vi "CRYDataView Curve Close.vi"   [LabVIEW 2013]
uses:
  CRYNew View Global.vi
types:
  T1 = typedef "Graph Main Info Cluster.ctl" = cluster{"Selected_BarIdx":i32, "Selected_PanelIdx":i32, "Graph Main VIRef":refnum<vi>, "ToolBarClick":bool, "Spliter Ref Array":refnum<vi>[], "Panel Ref Array":refnum<vi>[], "Spliter_matrix":i32[][], "Panel_matrix":i32[][], "child_spliterIdx_matrix":i32[][], "split_pos_matrix":i32[][], "Title State":bool, "sQueueName":string, "Frame nID":i32, "Graph VIRef Array":cluster{"Graph VIRef":refnum<vi>, "Panel Idx":i32, "Frame VIRef":refnum<vi>, "Icon Ring":i32, "Graph Type":string}[], "View Type":string}
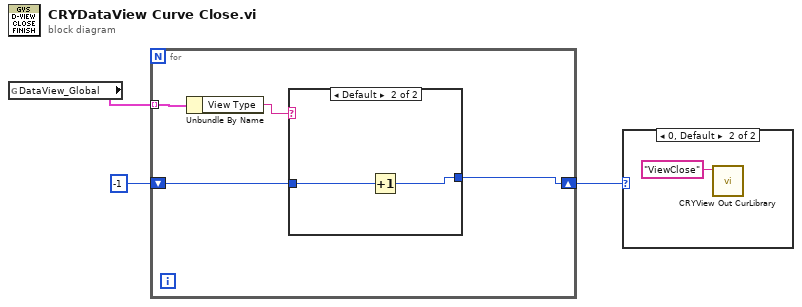
[diagram p0: block diagram]
diagram:
  n1 = global read "CRYNew View Global.vi" "DataView_Global"() -> (w3:T1[])
  n2 = for {
    tunnel: w3 -> [w7] mode=indexing
    shift-right: [w5] -> w1
    shift-left: -1 -> [w4]
    n3 = Unbundle By Name(w7) -> ("View Type"=w6:string)
    n4 = case shown="Default" w6 {
      tunnel: [w8 w9] -> w5
      tunnel: w4 -> [w8 w10]
      frame "ViewReport" {
      }
      frame Default {
        n5 = Increment(x=w10) -> (x+1=w9:i32)
      }
    }
  }
  n6 = case shown="0, Default" w1 {
    frame -1 {
    }
    frame 0, Default {
      n7 = call "CRYView Out CurLibrary.vi"("sAction"="ViewClose") -> ()  [unwired: 9 in, 2 out]
    }
  }
